vi "Arm Control.vi"(4 "Sally Door\nArm Position":dbl, 6 "Arm hic-up":dbl, 7 "Roller Speed":dbl=1.0, 8 "Arm Up":dbl, 9 "Arm down":dbl, 10 "Pot Value":dbl, 11 "Ball in Banner":bool) -> (0 "Current case":i32, 1 "Arm control method":i32, 2 "Roller Speed":dbl, 3 "Arm output":dbl)   [LabVIEW 2015]
panel:
  in  "Arm down":bool
  in  "Arm up":bool
  in  "Drawbridge":bool
  in  "Arm upper position":bool
  in  "Sally Door":bool
  in  "Harvest Button":bool
  # "Buttons"
  # "Sensors"
  # "Diagnostics"
  # "Setpoints"
  # "Outputs"
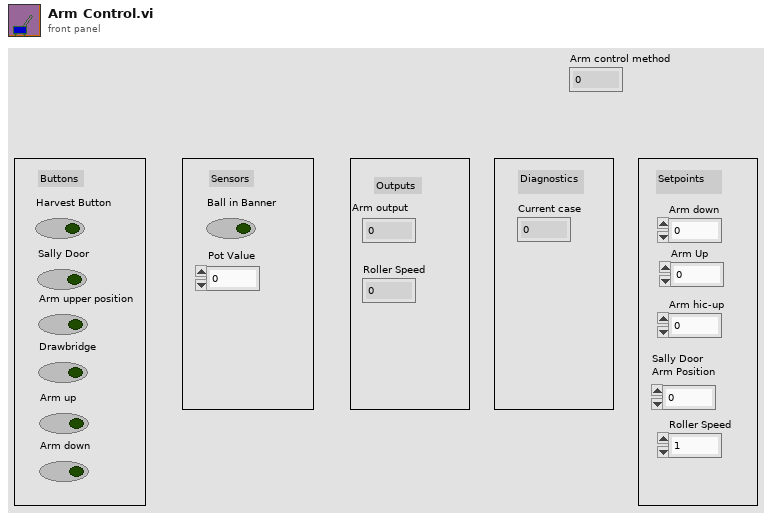
[diagram p1: front panel]
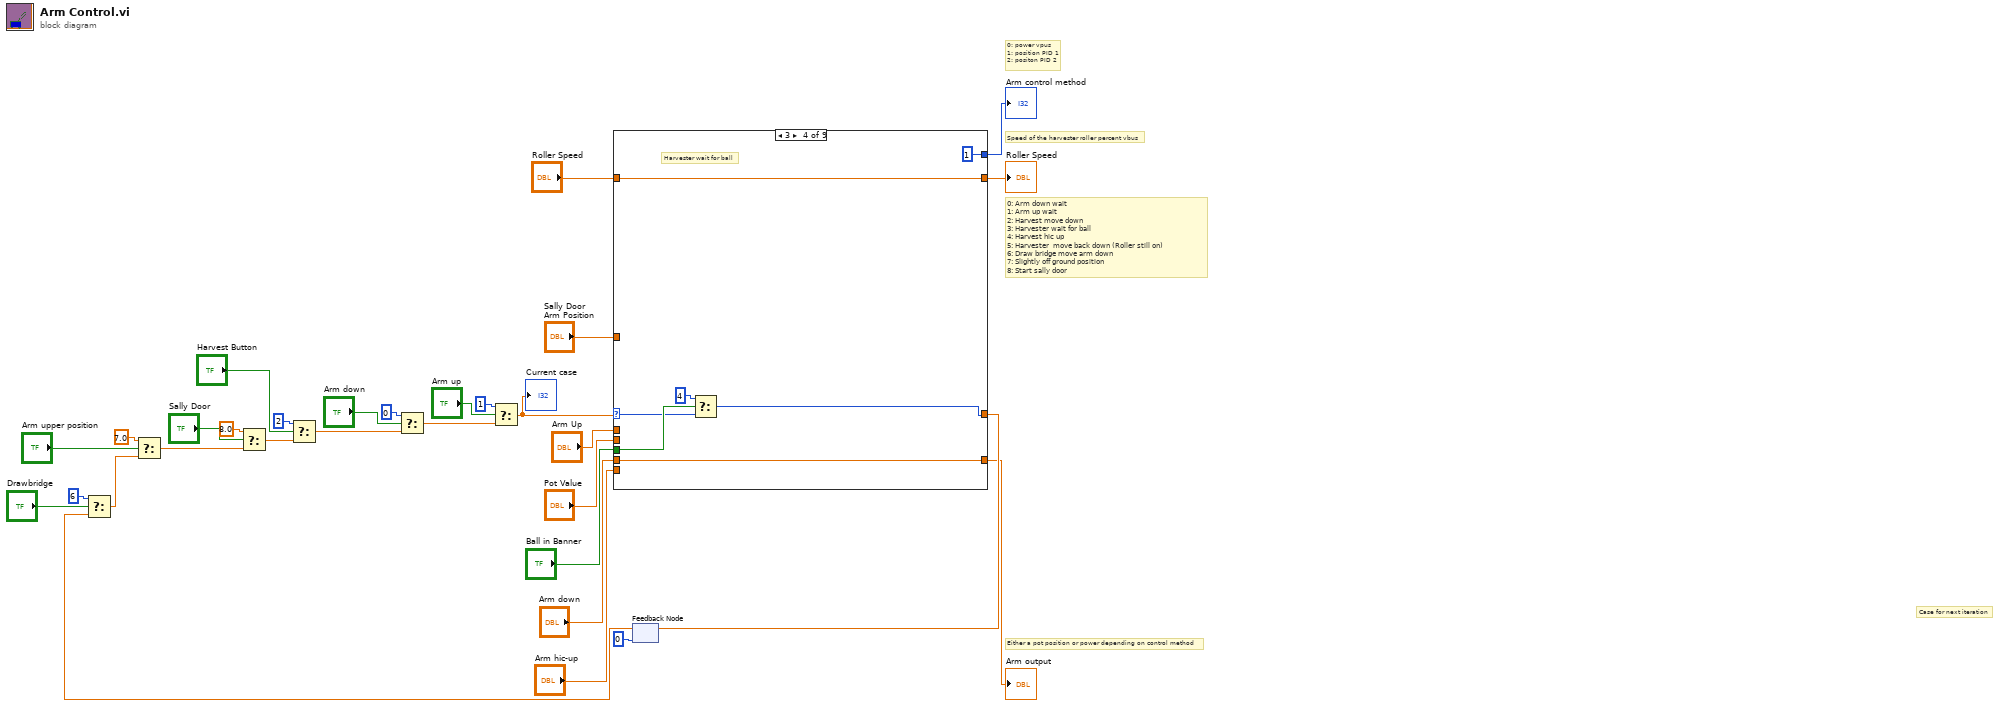
[diagram p0: block diagram]
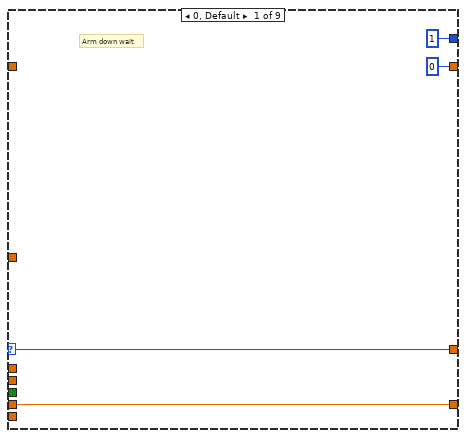
[diagram p2: hidden frame]
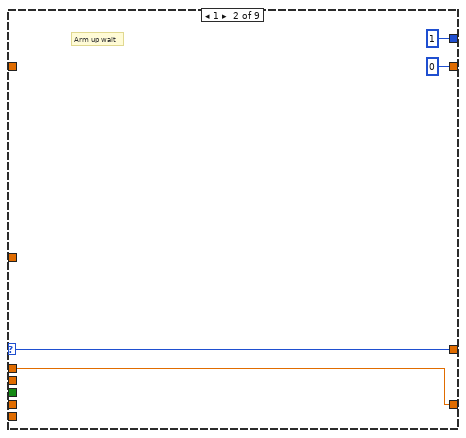
[diagram p3: hidden frame]
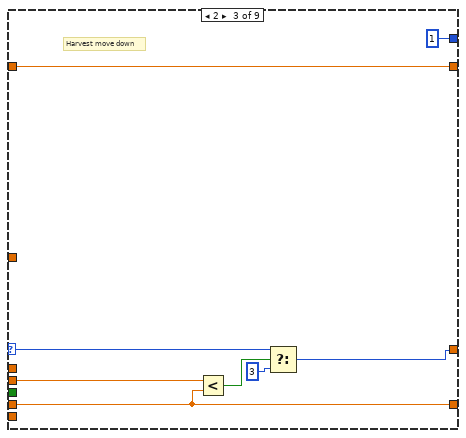
[diagram p4: hidden frame]
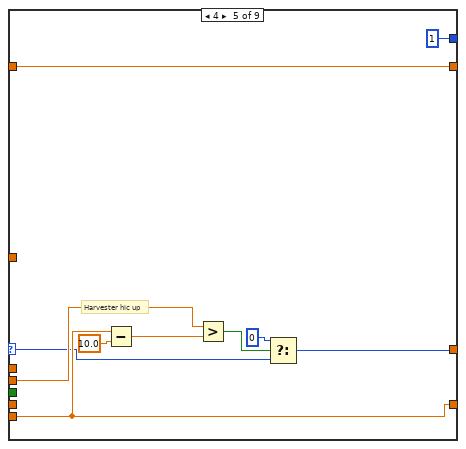
[diagram p5: hidden frame]
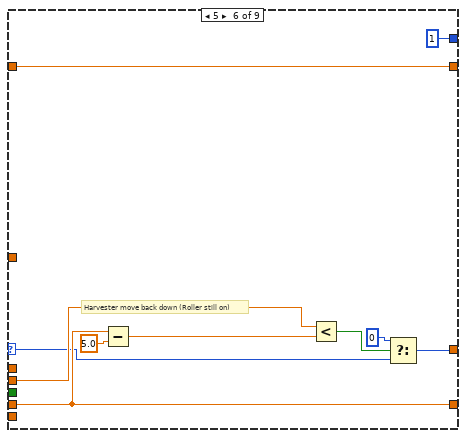
[diagram p6: hidden frame]
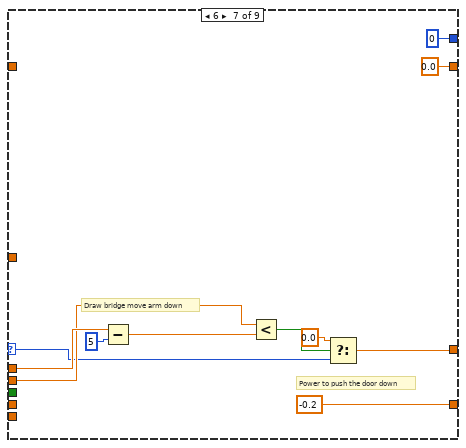
[diagram p7: hidden frame]
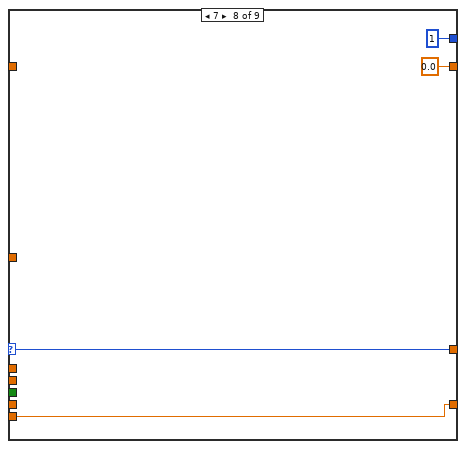
[diagram p8: hidden frame]
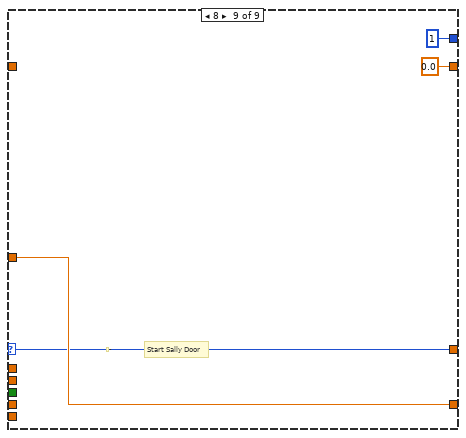
[diagram p9: hidden frame]
diagram:
  # "Case for next iteration"
  # "0: power vpus\n1: position PID 1\n2: positon PID 2"
  # "Speed of the harvester roller percent vbus"
  # "Either a pot position or power depending on control method"
  # "0: Arm down wait\n1: Arm up wait\n2: Harvest move down\n3: Harvester wait for ball\n4: Harvest hic up\n5: Harvester  move back down (Roller still on)\n6: Draw bridge move arm down\n7: Slightly off ground position\n8: Start sally door"
  n1 = feedback #1(0) -> (w6:dbl)
  n2 = Select(t=6, s="Drawbridge", f=w6) -> (s? t:f=w16:dbl)
  n3 = Select(t=7.0, s="Arm upper position", f=w16) -> (s? t:f=w15:dbl)
  n4 = Select(t=8.0, s="Sally Door", f=w15) -> (s? t:f=w14:dbl)
  n5 = Select(t=2, s="Harvest Button", f=w14) -> (s? t:f=w13:dbl)
  n6 = Select(t=0, s="Arm down", f=w13) -> (s? t:f=w12:dbl)
  n7 = Select(t=1, s="Arm up", f=w12) -> (s? t:f=w10:dbl)
  "Current case" <- w10
  n8 = case shown="3" w10 {
    selector: w10 -> [w33 w39 w42 w51 w58 w68 w76 w86 w91]
    tunnel: [w33 w39 w43 w49 w56 w67 w75 w86 w91] -> w31
    tunnel: "Pot Value" -> [_ _ w46 _ w59 w70 w79 _ _]
    tunnel: "Ball in Banner" -> [_ _ _ w52 _ _ _ _ _]
    tunnel: "Arm down" -> [w35 _ w44 w53 _ w73 _ _ _]
    tunnel: "Arm Up" -> [_ w38 _ _ _ _ w82 _ _]
    tunnel: "Arm hic-up" -> [_ _ _ _ w62 _ _ w89 _]
    tunnel: [w35 w38 w44 w53 w62 w73 -0.2 ("Arm down") w89 w93] -> w24
    tunnel: [0 0 w47 w54 w64 w74 0.0 ("Roller Speed") 0.0 ("Roller Speed") 0.0 ("Roller Speed")] -> w23
    tunnel: "Roller Speed" -> [_ _ w47 w54 w64 w74 _ _ _]
    tunnel: [1 1 1 1 1 1 0 1 1] -> w5
    tunnel: "Sally Door\nArm Position" -> [_ _ _ _ _ _ _ _ w93]
    frame 0, Default {
      # "Arm down wait"
    }
    frame 1 {
      # "Arm up wait"
    }
    frame 2 {
      # "Harvest move down"
      n9 = Less?(x=w46, y=w44) -> (x < y?=w45:bool)
      n10 = Select(t=w42, s=w45, f=3) -> (s? t:f=w43:i32)
    }
    frame 3 {
      # "Harvester wait for ball"
      n11 = Select(t=4, s=w52, f=w51) -> (s? t:f=w49:i32)
    }
    frame 4 {
      # "Harvester hic up"
      n12 = Subtract(x=w62, y=10.0) -> (x-y=w61:dbl)
      n13 = Greater?(x=w59, y=w61) -> (0:w63:bool)
      n14 = Select(t=0, s=w63, f=w58) -> (s? t:f=w56:i32)
    }
    frame 5 {
      # "Harvester move back down (Roller still on)"
      n15 = Subtract(x=w73, y=5.0) -> (x-y=w71:dbl)
      n16 = Less?(x=w70, y=w71) -> (x < y?=w69:bool)
      n17 = Select(t=0, s=w69, f=w68) -> (s? t:f=w67:i32)
    }
    frame 6 {
      # "Power to push the door down"
      # "Draw bridge move arm down"
      n18 = Subtract(x=w82, y=5) -> (x-y=w81:dbl)
      n19 = Less?(x=w79, y=w81) -> (x < y?=w78:bool)
      n20 = Select(t=0.0, s=w78, f=w76) -> (s? t:f=w75:dbl)
    }
    frame 7 {
    }
    frame 8 {
      # "-"
      # "Start Sally Door"
    }
  }
  "Arm output" <- w24
  "Roller Speed" <- w23
  "Arm control method" <- w5
  n21 = feedback-in #1(w31) -> ()
